vi "状态告警区.vi"(11 "数组":u16[](array[numeric]) format="%04xH") -> (3 "状态告警区":T1 {"告警代码" items=["无告警", "缺试剂告警", "缺水样告警", "缺蒸馏水告警", "缺标液告警", "仪表漏液告警", "标定异常告警", "超量程告警", "加热异常", "低试剂预警", "超上限告警", "超下限告警", "仪表内部其他异常", "滴定异常告警", "电极异常告警", "量程切换告警", "参数设置告警", "PH电极电位异常", "电导率电极异常", "浊度光度异常", "溶解氧电极异常", "溶解氧光强异常", "温度异常告警", "PH异常告警", "溶解氧异常告警", "电导率异常告警", "浊度异常告警", "叶绿素异常告警", "藻密度异常告警", "蓝绿藻异常告警", "ORP异常告警", "氨氮异常告警", "清洁刷异常告警", "SD卡异常告警", "蓝牙异常告警", "Wifi异常告警", "流程异常告警"]; "故障代码" items=["无故障", "电机故障", "温度故障", "通讯故障", "滴定故障"]})   [LabVIEW 2016, in "CODCr库.lvlib"]
panel:
  # "共占用24 WORD"
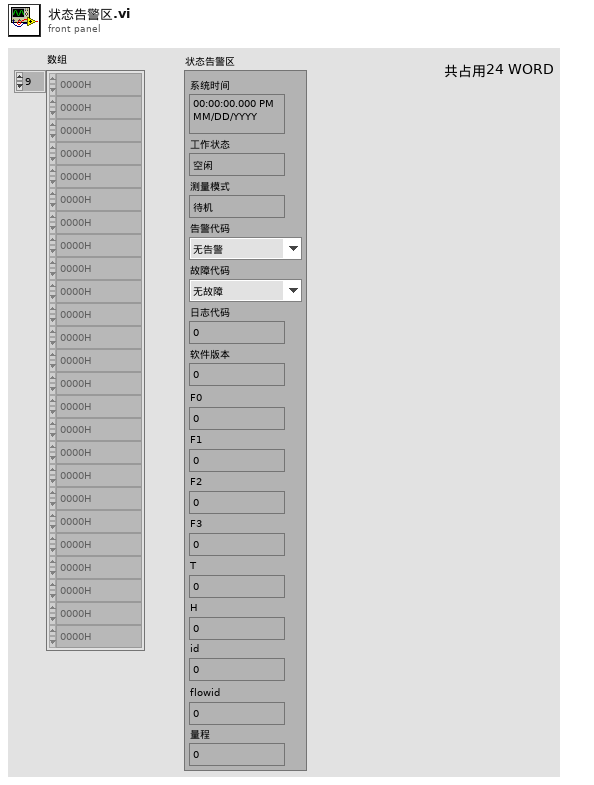
[diagram p1: front panel]
types:
  T1 = cluster{"系统时间":timestamp, "工作状态":enum16{"空闲", "水样测试", "标样核查", "零点核查", "跨度核查", "空白测试", "平行样测试", "加标回收", "空白校准", "标样校准", "初始化（清洗）"}, "测量模式":enum16{"待机", "连续模式", "周期模式", "定点模式", "受控模式", "手动模式"}, "告警代码":u16, "故障代码":u16, "日志代码":u16, "软件版本":u16, "F0":sgl, "F1":sgl, "F2":sgl, "F3":sgl, "T":sgl, "H":sgl, "id":u16, "flowid":u16, "量程":u16}
  T2 = cluster{"time stamp":timestamp, "WORD":u16, "WORD":u16, "WORD":u16, "WORD":u16, "WORD":u16, "WORD":u16, "FLOAT":sgl, "FLOAT":sgl, "FLOAT":sgl, "FLOAT":sgl, "FLOAT":sgl, "FLOAT":sgl, "WORD":u16, "WORD":u16, "WORD":u16}
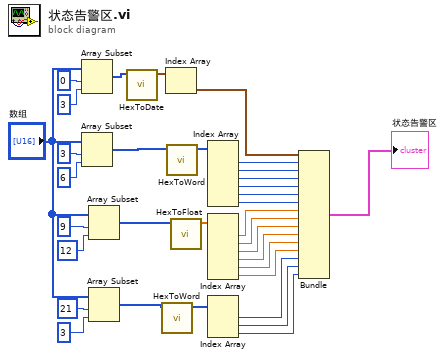
[diagram p0: block diagram]
diagram:
  n1 = Array Subset(array="数组", index=0 ("索引"), length=3 ("长度")) -> (w8:u16[])
  n2 = Array Subset(array="数组", index=3 ("索引"), length=6 ("长度")) -> (w6:u16[])
  n3 = Array Subset(array="数组", index=9 ("索引"), length=12 ("长度")) -> (w2:u16[])
  n4 = Array Subset(array="数组", index=21 ("索引"), length=3 ("索引")) -> (w4:u16[])
  n5 = call "HexToDate.vi"("数组"=w8) -> ("DATE"=w7:timestamp[])  [unwired: 10 in]
  n6 = call "HexToWord.vi"("数组"=w4) -> ("WORD"=w3:u16[])  [unwired: 10 in]
  n7 = Index Array(array=w7) -> (element=w30:timestamp)  [unwired: 1 in]
  n8 = call "HexToWord.vi"("数组"=w6) -> ("WORD"=w5:u16[])  [unwired: 10 in]
  n9 = call "HexToFloat.vi"("数组"=w2) -> ("FLOAT"=w1:sgl[])  [unwired: 10 in]
  n10 = Index Array(array=w5) -> (element #1=w29:u16, element #2=w28:u16, element #3=w27:u16, element #4=w26:u16, element #5=w25:u16, element #6=w24:u16)  [unwired: 6 in]
  n11 = Index Array(array=w1) -> (element #1=w21:sgl, element #2=w20:sgl, element #3=w19:sgl, element #4=w18:sgl, element #5=w17:sgl, element #6=w16:sgl)  [unwired: 6 in]
  n12 = Index Array(array=w3) -> (element #1=w12:u16, element #2=w11:u16, element #3=w10:u16)  [unwired: 3 in]
  n13 = Bundle("time stamp"=w30, "WORD"=w29, "WORD"=w28, "WORD"=w27, "WORD"=w26, "WORD"=w25, "WORD"=w24, "FLOAT"=w21, "FLOAT"=w20, "FLOAT"=w19, "FLOAT"=w18, "FLOAT"=w17, "FLOAT"=w16, "WORD"=w12, "WORD"=w11, "WORD"=w10) -> (→"状态告警区":T2)  [unwired: 1 in]
